vi "array to vision.vi"(8 "error in (no error)":errorcluster, 11 "Thorcam in":refnum<class "Thorcam.lvclass">) -> (0 "error out":errorcluster, 3 "Thorcam out":refnum<class "Thorcam.lvclass">)   [LabVIEW 2012, in "Thorcam.lvclass"]
uses:
  Thorcam.lvclass
  Thorcam.lvclass/Thorcam.ctl
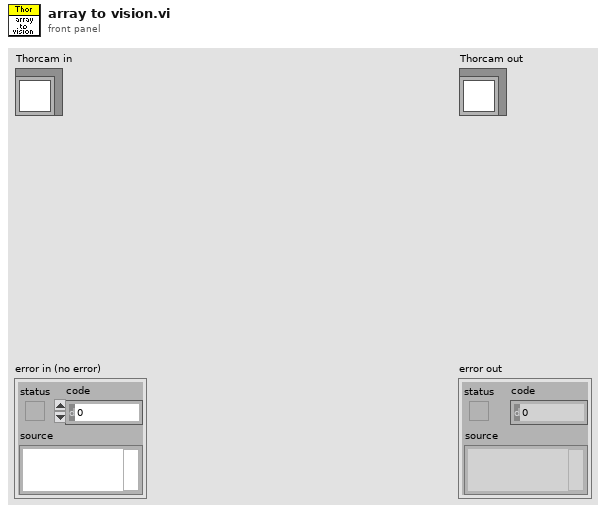
[diagram p1: front panel]
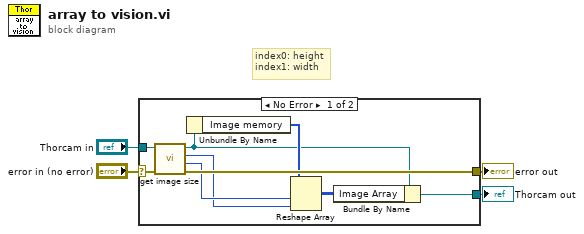
[diagram p0: block diagram]
diagram:
  # "index0: height\nindex1: width"
  n1 = case shown="No Error" "error in (no error)" {
    selector: "error in (no error)" -> [w13 w15]
    tunnel: [w12 w15] -> w3
    tunnel: [w8 w14] -> w1
    tunnel: "Thorcam in" -> [w11 w14]
    frame No Error {
      n2 = call-dynamic "get image size.vi"("error in (no error)"=w13, "Thorcam in"=w11) -> ("error out"=w12:errorcluster, "Height"=w7:i32, "Width"=w6:i32, "Thorcam out"=w9:refnum<class "Thorcam.lvclass">)  [unwired: 6 in]
      n3 = Unbundle By Name(w9) -> ("Image memory"=w10:u8[])
      n4 = Reshape Array(w10, w7, w6) -> (w5:u8[][])
      n5 = Bundle By Name(cluster=w9, "Image Array"=w5) -> (w8:refnum<class "Thorcam.lvclass">)
    }
    frame Error {
    }
  }
  "error out" <- w3
  "Thorcam out" <- w1
